vi "Picture matching.vi"() -> ()   [LabVIEW 2018]
uses:
  <vilib>/userdefined/High Color/IMAQdx.ctl
  <vilib>/vision/driver/NI_Vision_Acquisition_Software.lvlib
  <vilib>/vision/NI_Vision_Development_Module.lvlib
panel:
  in  "stop":bool
  out "error out 2":errorcluster
  out "Tamplate":T1(plugin-control)
  out "Image":T1(plugin-control)
  in  "Parameters":T2={"Number of Matches Requested"=1, "Minimum Match Score"=800.0, "Angle Ranges"=[]}
  in  "File Path":path
  out "error out":errorcluster
  in  "Session In":T3
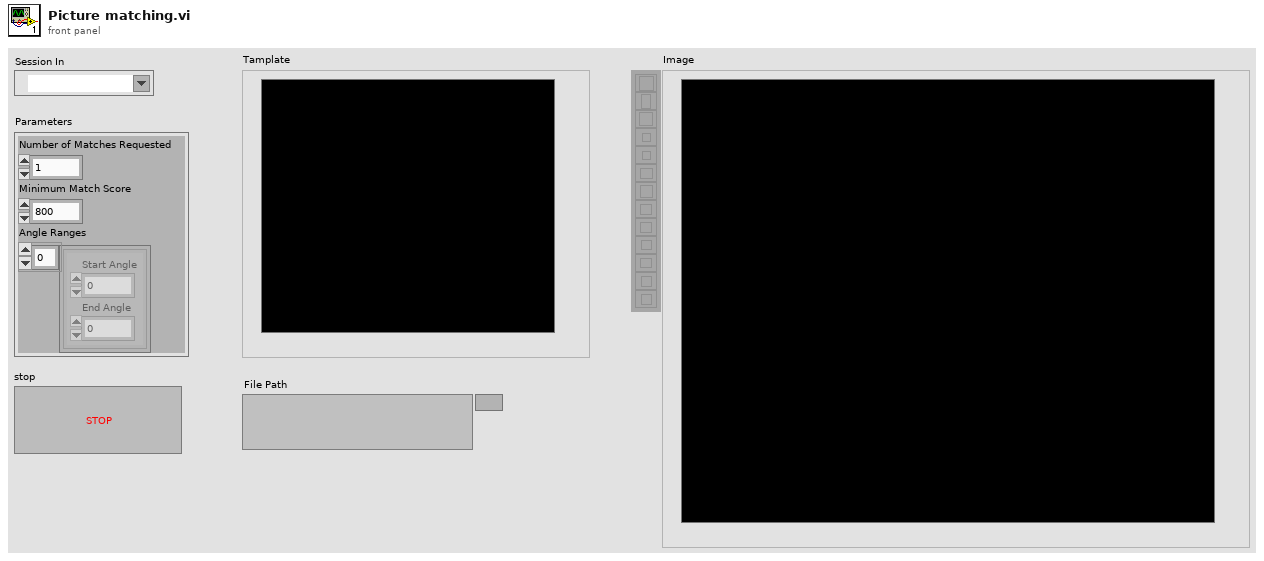
[diagram p1: front panel]
types:
  T1 = typedef "IMAQ Image.ctl" = refnum<image>
  T2 = cluster{"Number of Matches Requested":i32, "Minimum Match Score":sgl, "Angle Ranges":cluster{"Start Angle":sgl, "End Angle":sgl}[]}
  T3 = typedef "IMAQdx.ctl" = refnum<k21>
  T4 = cluster{"Position":cluster{"x":sgl, "y":sgl}, "Angle":sgl, "Scale":sgl, "Score":sgl, "Bounding Box":cluster{"x":sgl, "y":sgl}[]}[]
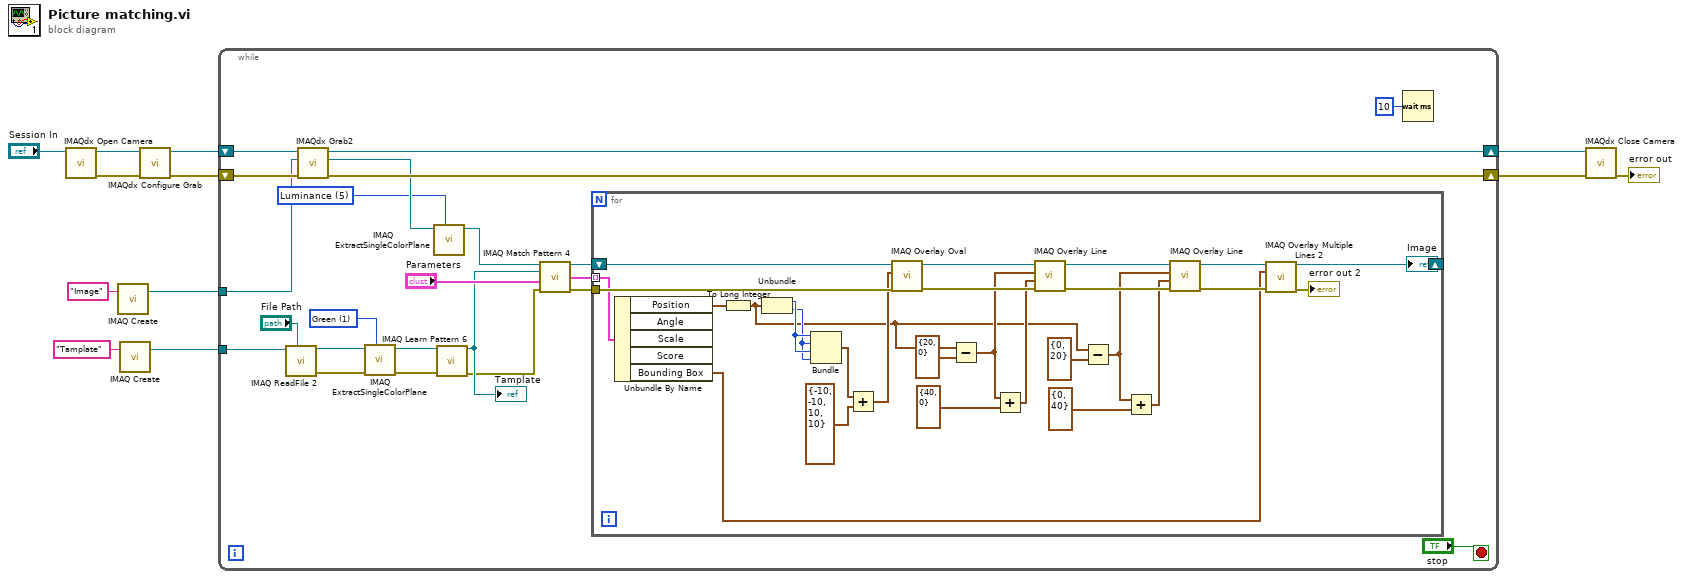
[diagram p0: block diagram]
diagram:
  n1 = call <vilib>:"IMAQdx Open Camera.vi"("Session In"="Session In") -> ("error out"=w10:errorcluster, "Session Out"=w11:T3)  [unwired: 9 in]
  n2 = call "IMAQ Create"("Image Name"="Image") -> ("New Image"=w1:T1)  [unwired: 4 in, 1 out]
  n3 = call "IMAQ Create"("Image Name"="Tamplate") -> ("New Image"=w5:T1)  [unwired: 4 in, 1 out]
  n4 = call <vilib>:"IMAQdx Configure Grab.vi"("error in"=w10, "Session In"=w11) -> ("error out"=w3:errorcluster, "Session Out"=w4:T3)  [unwired: 8 in]
  n5 = while {
    shift-right: [w33] -> w9
    shift-left: w4 -> [w35]
    shift-right: [w32] -> w8
    shift-left: w3 -> [w34]
    tunnel: w5 -> [w36]
    tunnel: w1 -> [w31]
    stop <- "stop" stop-if-true
    w13 = 1 items=["Red", "Green", "Blue", "Hue", "Saturation", "Luminance", "Value", "Intensity"] ("Color Plane")
    w20 = 5 items=["Red", "Green", "Blue", "Hue", "Saturation", "Luminance", "Value", "Intensity"] ("Color Plane")
    n6 = call "IMAQ ReadFile 2"("File Path"="File Path", "Image"=w36) -> ("error out"=w16:errorcluster, "Image Out"=w14:T1)  [unwired: 5 in, 3 out]
    n7 = call <vilib>:"IMAQdx Grab2.vi"("error in"=w34, "Image In"=w31, "Session In"=w35) -> ("error out"=w32:errorcluster, "Image Out"=w21:T1, "Session Out"=w33:T3)  [unwired: 5 in, 1 out]
    n8 = call "IMAQ ExtractSingleColorPlane"("Color Plane"=w13, "error in (no error)"=w16, "Image Src"=w14) -> ("error out"=w15:errorcluster, "Image Dst Out"=w17:T1)  [unwired: 7 in]
    n9 = call "IMAQ ExtractSingleColorPlane"("Color Plane"=w20, "Image Src"=w21) -> ("Image Dst Out"=w19:T1)  [unwired: 8 in, 1 out]
    n10 = call "IMAQ Learn Pattern 6"("Image"=w17, "error in (no error)"=w15) -> ("Template Image Out"=w28:T1, "error out"=w24:errorcluster)  [unwired: 11 in, 1 out]
    "Tamplate" <- w28
    n11 = call "IMAQ Match Pattern 4"("Image"=w19, "Template Image"=w28, "Parameters"="Parameters", "error in (no error)"=w24) -> ("Image (duplicate)"=w27:T1, "Matches (real-world)"=w23:T4, "error out"=w25:errorcluster)  [unwired: 7 in, 2 out]
    n12 = for {
      tunnel: w25 -> [w58]
      shift-right: [w59] -> w26
      shift-left: w27 -> [w63]
      tunnel: w23 -> [w54] mode=indexing
      n13 = Unbundle By Name(w54) -> ("Position"=w53:cluster{"x":sgl, "y":sgl}, "Bounding Box"=w50:cluster{"x":sgl, "y":sgl}[])  [unwired: 3 out]
      n14 = To Long Integer(number=w53) -> (32bit integer=w39:cluster{"x":i32, "y":i32})
      n15 = Unbundle(w39) -> ("x"=w52:i32, "y"=w51:i32)
      n16 = Bundle("x"=w52, "y"=w51, "x"=w52, "y"=w51) -> (w48:cluster{"x":i32, "y":i32, "x":i32, "y":i32})  [unwired: 1 in]
      n17 = Add(x=w48, y=cluster{"x":i32, "y":i32, "x":i32, "y":i32} {"x"=-10, "y"=-10, "x"=10, "y"=10}) -> (x+y=w47:cluster{"x":i32, "y":i32, "x":i32, "y":i32})
      n18 = call "IMAQ Overlay Oval"("error in (no error)"=w58, "Bounding Rectangle"=w47, "Image"=w63) -> ("error out"=w57:errorcluster, "Image Out"=w62:T1)  [unwired: 7 in]
      n19 = Subtract(x=w39, y=cluster{"x":i32, "y":i32} {"x"=20, "y"=0}) -> (x-y=w43:cluster{"x":i32, "y":i32})
      n20 = Add(x=w43, y=cluster{"x":i32, "y":i32} {"x"=40, "y"=0}) -> (x+y=w42:cluster{"x":i32, "y":i32})
      n21 = call "IMAQ Overlay Line"("error in (no error)"=w57, "End Point"=w42, "Start Point"=w43, "Image"=w62) -> ("error out"=w56:errorcluster, "Image Out"=w61:T1)  [unwired: 6 in]
      n22 = Subtract(x=w39, y=cluster{"x":i32, "y":i32} {"x"=0, "y"=20}) -> (x-y=w38:cluster{"x":i32, "y":i32})
      n23 = Add(x=w38, y=cluster{"x":i32, "y":i32} {"x"=0, "y"=40}) -> (x+y=w37:cluster{"x":i32, "y":i32})
      n24 = call "IMAQ Overlay Line"("error in (no error)"=w56, "End Point"=w37, "Start Point"=w38, "Image"=w61) -> ("error out"=w55:errorcluster, "Image Out"=w60:T1)  [unwired: 6 in]
      n25 = call "IMAQ Overlay Multiple Lines 2"("Image"=w60, "Line End Points"=w50, "error in (no error)"=w55) -> ("Image Out"=w59:T1, "error out"=→"error out 2":errorcluster)  [unwired: 11 in]
    }
    "Image" <- w26
    n26 = Wait (ms)(milliseconds to wait=u32 10) -> ()  [unwired: 1 out]
  }
  n27 = call <vilib>:"IMAQdx Close Camera.vi"("error in"=w8, "Session In"=w9) -> ("error out"=→"error out":errorcluster)  [unwired: 9 in]
